vi "Game_Main.vi"(8 "error in (no error)":errorcluster, 10 "Players array":T1[](array[typedef]), 11 "Queue Bus":T2) -> (0 "error out":errorcluster)   [LabVIEW 2020]
uses:
  Typedefs/queueBus.ctl
  Typedefs/communicationData.ctl
  Typedefs/game_player.ctl
  Typedefs/enumeratedPlayers.ctl
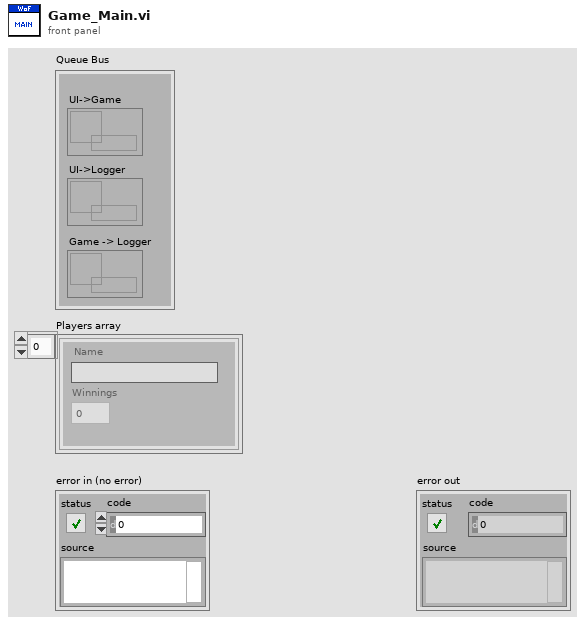
[diagram p1: front panel]
types:
  T1 = typedef "game_player.ctl" = cluster{"Name":string, "Winnings":dbl}
  T2 = typedef "queueBus.ctl" = cluster{"UI->Game":refnum<queue>, "UI->Logger":refnum<queue>, "Game -> Logger":refnum<queue>}
  T3 = typedef "enumeratedPlayers.ctl" = enum16{"one", "two", "three"}
  T4 = typedef "communicationData.ctl" = cluster{"command":string, "payload":variant, "response":variant}
  T5 = typedef "gameState.ctl" = cluster{"active player":T3, "Winnings":dbl[], "Vowel Enabled?":bool, "Puzzle State":string, "Puzzle Solved?":bool}
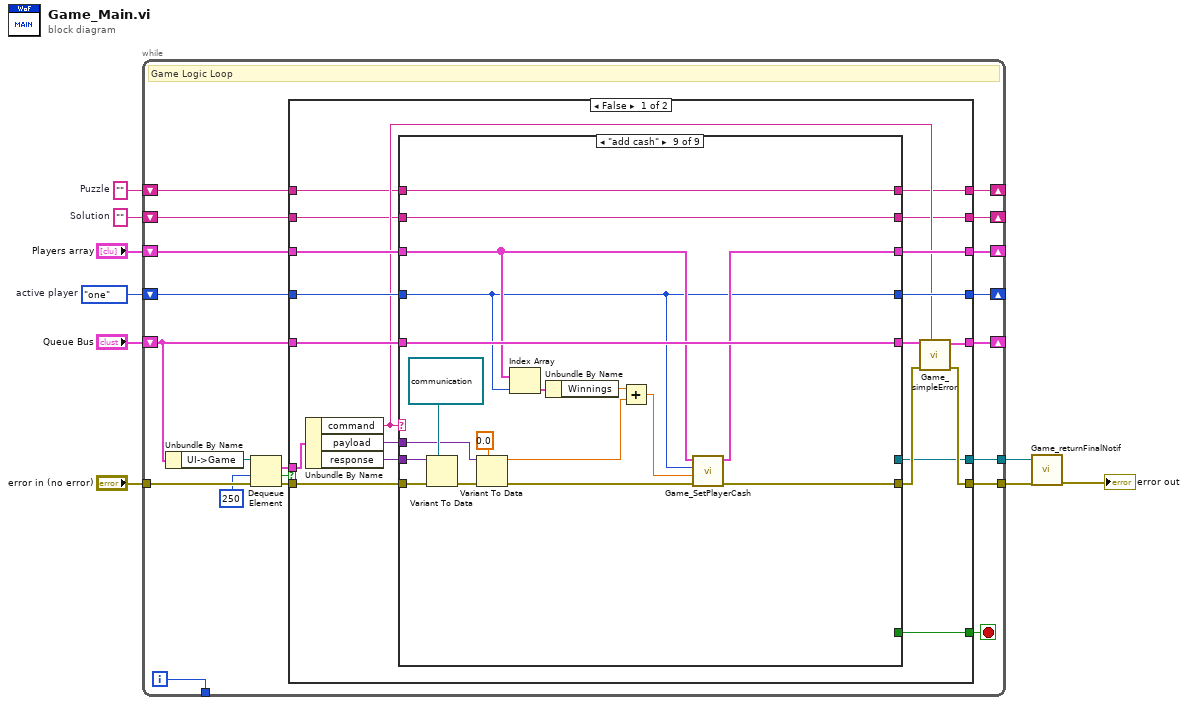
[diagram p0: block diagram]
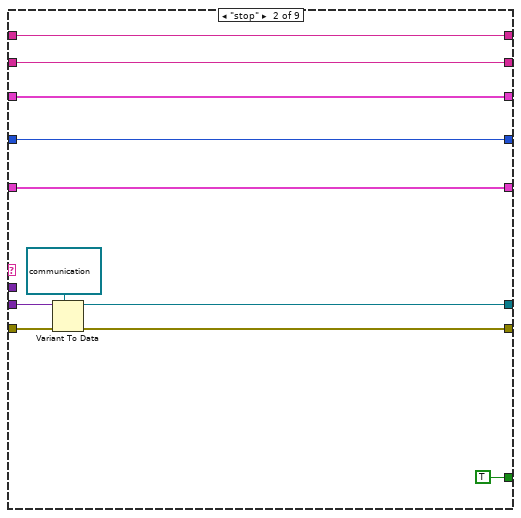
[diagram p3: hidden frame]
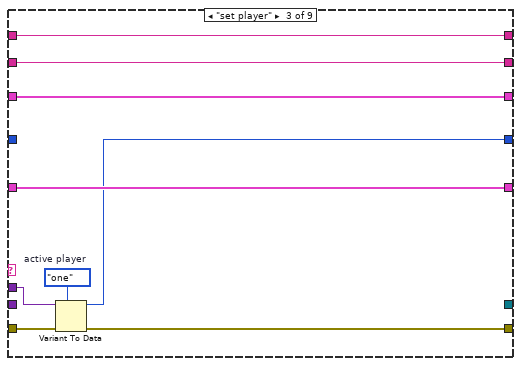
[diagram p4: hidden frame]
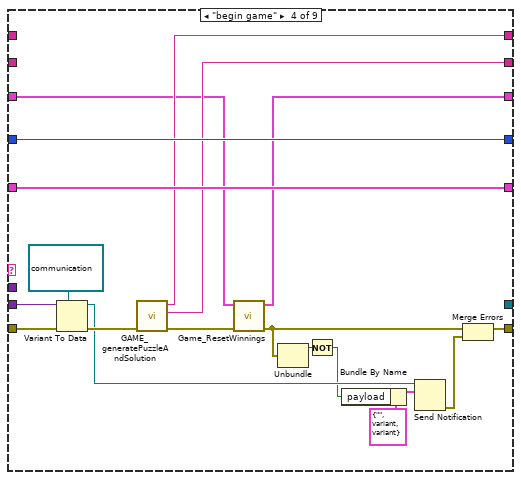
[diagram p5: hidden frame]
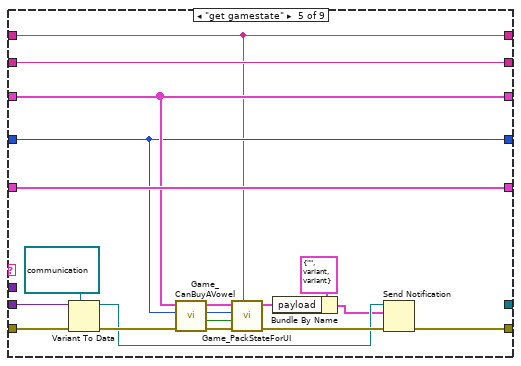
[diagram p6: hidden frame]
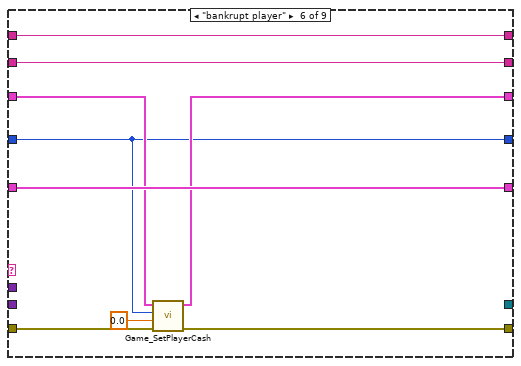
[diagram p7: hidden frame]
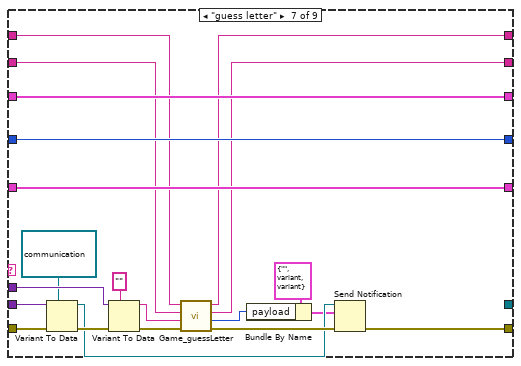
[diagram p8: hidden frame]
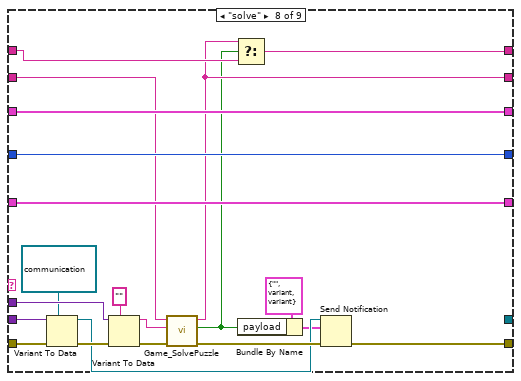
[diagram p9: hidden frame]
diagram:
  w1 = ""  # Solution
  w2 = ""  # Puzzle
  w6 = enumeratedPlayers."one"  # active player
  n1 = while {
    shift-right: [w22] -> _
    shift-left: "Queue Bus" -> [w23]
    tunnel: "error in (no error)" -> [w29]
    shift-right: [w20] -> _
    shift-left: "Players array" -> [w21]
    shift-right: [w18] -> _
    shift-left: w6 -> [w19]
    tunnel: [w16] -> w5
    tunnel: [w15] -> w3
    tunnel: [w14] -> _
    shift-right: [w11] -> _
    shift-left: w2 -> [w13]
    shift-right: [w10] -> _
    shift-left: w1 -> [w12]
    i -> [w14]
    stop <- w17 stop-if-true
    # "Game Logic Loop"
    n2 = Unbundle By Name(w23) -> ("UI->Game"=w28:refnum<queue>)
    n3 = Dequeue Element(queue=w28, timeout in ms (-1)=250, error in (no error)=w29) -> (element=w24:T4, timed out?=w26:bool, error out=w25:errorcluster)  [unwired: 1 out]
    n4 = case shown="False" w26 {
      tunnel: w25 -> [w44 w185]
      tunnel: w24 -> [w47 _]
      tunnel: w23 -> [w43 w188]
      tunnel: [w35 w188] -> w22
      tunnel: w21 -> [w42 w187]
      tunnel: [w41 w187] -> w20
      tunnel: w19 -> [w40 w186]
      tunnel: [w39 w186] -> w18
      tunnel: [w38 _] -> w17
      tunnel: [w48 w185] -> w16
      tunnel: [w37 _] -> w15
      tunnel: w13 -> [w33 w184]
      tunnel: w12 -> [w32 w183]
      tunnel: [w31 w184] -> w11
      tunnel: [w30 w183] -> w10
      frame False {
        n5 = Unbundle By Name(w47) -> ("command"=w34:string, "payload"=w46:variant, "response"=w45:variant)
        n6 = case shown="\"add cash\"" w34 {
          tunnel: w46 -> [_ _ w71 _ _ _ w139 w159 w175]
          tunnel: w45 -> [_ w62 _ w85 w101 _ w129 w156 w177]
          tunnel: w44 -> [w52 w63 w73 w92 w112 w119 w140 w160 w181]
          tunnel: w43 -> [w55 w66 w75 w94 w113 w122 w143 w163 w182]
          tunnel: [w55 w66 w75 w94 w113 w122 w143 w163 w182] -> w36
          tunnel: w42 -> [w54 w65 w74 w88 w110 w117 w142 w162 w168]
          tunnel: [w54 w65 w74 w87 w110 w116 w142 w162 w167] -> w41
          tunnel: w40 -> [w53 w64 _ w93 w109 w115 w141 w161 w165]
          tunnel: [w53 w64 w69 w93 w109 w115 w141 w161 w165] -> w39
          tunnel: [_ TRUE _ _ _ _ _ _ _] -> w38
          tunnel: [w52 w59 w72 w77 w99 w118 w127 w154 w169] -> w49
          tunnel: [_ w58 _ _ _ _ _ _ _] -> w37
          tunnel: w33 -> [w51 w57 w68 _ w103 w121 w133 w147 w180]
          tunnel: w32 -> [w50 w56 w67 _ w111 w120 w134 w148 w179]
          tunnel: [w51 w57 w68 w91 w103 w121 w132 w144 w180] -> w31
          tunnel: [w50 w56 w67 w90 w111 w120 w131 w146 w179] -> w30
          frame Default {
          }
          frame "stop" {
            n7 = Variant To Data(error in=w63, type=refnum<notifier> refnum ("notifier out"), Variant=w62) -> (data=w58:refnum<notifier>, error out=w59:errorcluster)
          }
          frame "set player" {
            w70 = enumeratedPlayers."one"  # active player
            n8 = Variant To Data(error in=w73, type=w70, Variant=w71) -> (data=w69:T3, error out=w72:errorcluster)
          }
          frame "begin game" {
            n9 = Variant To Data(error in=w92, type=refnum<notifier> refnum ("notifier out"), Variant=w85) -> (data=w81:refnum<notifier>, error out=w86:errorcluster)
            n10 = call "GAME_generatePuzzleAndSolution.vi"("error in (no error)"=w86) -> ("error out"=w89:errorcluster, "Solution"=w90:string, "Puzzle"=w91:string)  [unwired: 8 in]
            n11 = call "Game_ResetWinnings.vi"("error in (no error)"=w89, "Players array"=w88) -> ("error out"=w83:errorcluster, "Players array OUT"=w87:T1[])  [unwired: 8 in]
            n12 = Unbundle(w83) -> ("status"=w82:bool)  [unwired: 2 out]
            n13 = Not(x=w82) -> (.not. x?=w78:bool)
            n14 = Bundle By Name(cluster=T4 {"command"="", "payload"=variant, "response"=variant} ("notification"), "payload"=w78) -> (w79:T4)
            n15 = Send Notification(notification=w79, notifier=w81) -> (error out=w76:errorcluster)  [unwired: 1 in, 1 out]
            n16 = Merge Errors(w83, w76) -> (w77:errorcluster)
          }
          frame "get gamestate" {
            n17 = Variant To Data(error in=w112, type=refnum<notifier> refnum ("notifier out"), Variant=w101) -> (data=w98:refnum<notifier>, error out=w102:errorcluster)
            n18 = call "Game_CanBuyAVowel.vi"("error in (no error)"=w102, "player"=w109, "Players array"=w110) -> ("error out"=w108:errorcluster, "CanBuy?"=w104:bool, "player OUT"=w105:T3, "Players array OUT"=w106:T1[])  [unwired: 5 in]
            n19 = call "Game_PackStateForUI.vi"("Puzzle State"=w103, "error in (no error)"=w108, "Can Buy Vowel?"=w104, "player"=w105, "Players array"=w106) -> ("error out"=w107:errorcluster, "gameState"=w96:T5)  [unwired: 5 in]
            n20 = Bundle By Name(cluster=T4 {"command"="", "payload"=variant, "response"=variant} ("notification"), "payload"=w96) -> (w95:T4)
            n21 = Send Notification(notification=w95, notifier=w98, error in (no error)=w107) -> (error out=w99:errorcluster)  [unwired: 1 out]
          }
          frame "bankrupt player" {
            n22 = call "Game_SetPlayerCash.vi"("error in (no error)"=w119, "Amount"=0.0, "player"=w115, "Players array"=w117) -> ("error out"=w118:errorcluster, "Players array OUT"=w116:T1[])  [unwired: 6 in]
          }
          frame "guess letter" {
            n23 = Variant To Data(error in=w140, type=refnum<notifier> refnum ("notifier out"), Variant=w129) -> (data=w126:refnum<notifier>, error out=w130:errorcluster)
            n24 = Variant To Data(error in=w130, type="", Variant=w139) -> (data=w135:string, error out=w137:errorcluster)
            n25 = call "Game_guessLetter.vi"("error in (no error)"=w137, "guess"=w135, "Solution"=w134, "Puzzle"=w133) -> ("error out"=w136:errorcluster, "Letters Found"=w124:i32, "Solution OUT"=w131:string, "Puzzle OUT"=w132:string)  [unwired: 4 in]
            n26 = Bundle By Name(cluster=T4 {"command"="", "payload"=variant, "response"=variant} ("notification"), "payload"=w124) -> (w123:T4)
            n27 = Send Notification(notification=w123, notifier=w126, error in (no error)=w136) -> (error out=w127:errorcluster)  [unwired: 1 out]
          }
          frame "solve" {
            n28 = Variant To Data(error in=w160, type=refnum<notifier> refnum ("notifier out"), Variant=w156) -> (data=w153:refnum<notifier>, error out=w157:errorcluster)
            n29 = Variant To Data(error in=w157, type="", Variant=w159) -> (data=w149:string, error out=w150:errorcluster)
            n30 = call "Game_SolvePuzzle.vi"("error in (no error)"=w150, "Guess"=w149, "Solution"=w148) -> ("error out"=w164:errorcluster, "Correct"=w145:bool, "Solution OUT"=w146:string)  [unwired: 6 in]
            n31 = Select(t=w146, s=w145, f=w147) -> (s? t:f=w144:string)
            n32 = Bundle By Name(cluster=T4 {"command"="", "payload"=variant, "response"=variant} ("notification"), "payload"=w145) -> (w151:T4)
            n33 = Send Notification(notification=w151, notifier=w153, error in (no error)=w164) -> (error out=w154:errorcluster)  [unwired: 1 out]
          }
          frame "add cash" {
            n34 = Variant To Data(error in=w181, type=refnum<notifier> refnum ("notifier out"), Variant=w177) -> (error out=w178:errorcluster)  [unwired: 1 out]
            n35 = Variant To Data(error in=w178, type=0.0, Variant=w175) -> (data=w172:dbl, error out=w170:errorcluster)
            n36 = Index Array(array=w168, index=w165) -> (element=w173:T1)
            n37 = Unbundle By Name(w173) -> ("Winnings"=w171:dbl)
            n38 = Add(x=w171, y=w172) -> (x+y=w166:dbl)
            n39 = call "Game_SetPlayerCash.vi"("error in (no error)"=w170, "Amount"=w166, "player"=w165, "Players array"=w168) -> ("error out"=w169:errorcluster, "Players array OUT"=w167:T1[])  [unwired: 6 in]
          }
        }
        n40 = call "Game_simpleError.vi"("command"=w34, "error in (no error)"=w49, "Queue Bus"=w36) -> ("error out"=w48:errorcluster, "Queue Bus OUT"=w35:T2)  [unwired: 7 in]
      }
      frame True {
      }
    }
  }
  n41 = call "Game_returnFinalNotif.vi"("error in (no error)"=w5, "notifier"=w3) -> ("error out"=→"error out":errorcluster)  [unwired: 9 in]
